vi "set_lens_NA.vi"(8 "error in (no error)":errorcluster, 10 "lens NA":dbl, 11 "GenericObjective in":refnum<class "GenericObjective.lvclass">) -> (0 "error out":errorcluster, 3 "GenericObjective out":refnum<class "GenericObjective.lvclass">)   [LabVIEW 2010, in "GenericObjective.lvclass"]
uses:
  GenericObjective.lvclass
  GenericObjective.lvclass/GenericObjective.ctl
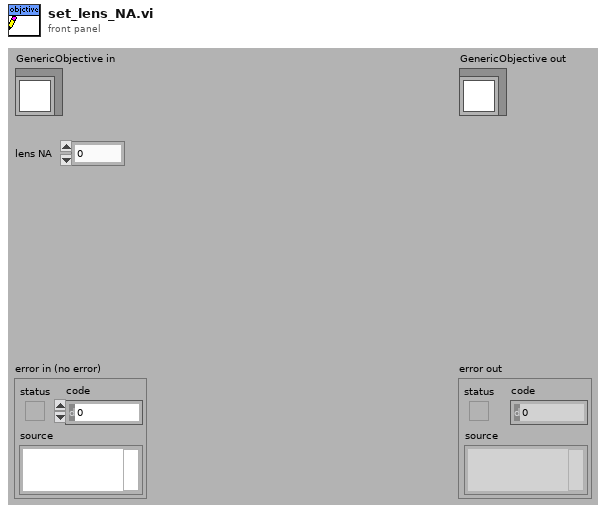
[diagram p1: front panel]
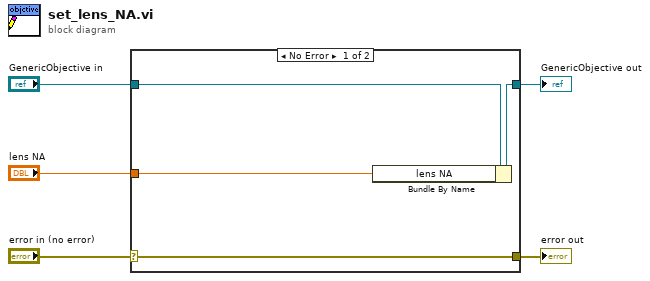
[diagram p0: block diagram]
diagram:
  n1 = case shown="No Error" "error in (no error)" {
    selector: "error in (no error)" -> [w9 w10]
    tunnel: [w9 w10] -> w4
    tunnel: [w7 w11] -> w2
    tunnel: "GenericObjective in" -> [w8 w11]
    tunnel: "lens NA" -> [w6 _]
    frame No Error {
      n2 = Bundle By Name(cluster=w8, "lens NA"=w6) -> (w7:refnum<class "GenericObjective.lvclass">)
    }
    frame Error {
    }
  }
  "error out" <- w4
  "GenericObjective out" <- w2
